vi "Read Dependencies.vi"(8 "error in (no error)":errorcluster, 11 "Selection in":refnum<class "Selection.lvclass">) -> (0 "error out":errorcluster, 2 "Dependencies":refnum<data-value>[](array[refnum]), 3 "Selection out":refnum<class "Selection.lvclass">)   [LabVIEW 2017, in "LV Image Editor Framework.lvlib" / "Selection.lvclass"]
uses:
  Selection.lvclass
  Shape/Shape.lvclass
  Selection.lvclass/Selection.ctl
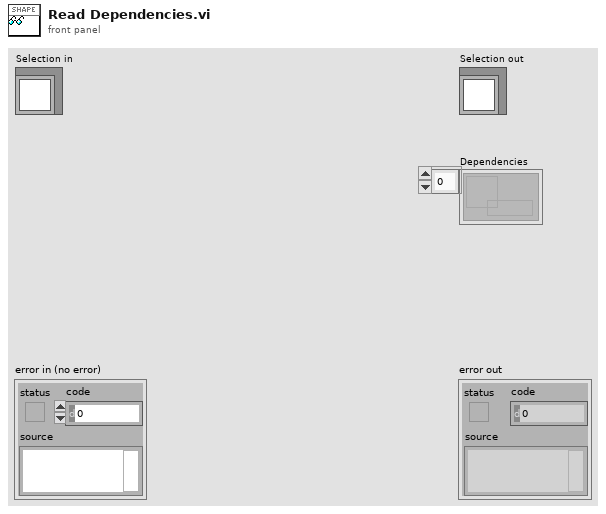
[diagram p1: front panel]
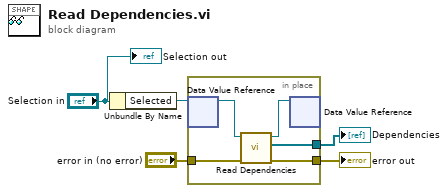
[diagram p0: block diagram]
diagram:
  n1 = Unbundle By Name("Selection in") -> ("Selected"=w4:refnum<data-value>)
  n2 = in-place {
    in-place-border: "error in (no error)" -> [w10]
    in-place-border: [w7] -> w2
    in-place-border: [w6] -> w1
    n3 = in-place-dvr #1(w4) -> (w9:refnum<class "Shape.lvclass">)  [unwired: 1 out]
    n4 = call-dynamic "Read Dependencies.vi"("error in (no error)"=w10, "Shape in"=w9) -> ("error out"=w7:errorcluster, "Dependencies"=w6:refnum<data-value>[], "Shape out"=w8:refnum<class "Shape.lvclass">)  [unwired: 7 in]
    n5 = in-place-dvr #1(w8) -> ()  [unwired: 2 out]
  }
  "error out" <- w2
  "Dependencies" <- w1
  "Selection out" <- "Selection in"
